vi "抓圓.vi"(0 "Image In":T2, 1 "Process":T7(ring), 2 "Optimized Mode":bool, 3 "Direction":enum16{"Inner to Outer", "Outer to Inner"}(ring), 5 "ROI":T1, 9 "Gap":i32=10 min=1 max=300, 11 "error In":errorcluster, 12 "Edge Options":T5={"Edge Polarity"=0, "Kernel Size"=3, "Width"=3, "Minimum Edge Strength"=10.0, "Interpolation Type"=enum."Bilinear Fixed", "Data Processing Method"=enum."Average"} {"Edge Polarity" items=["All Edges", "Rising Edges", "Falling Edges"]; "Minimum Edge Strength" format="%.2f"; "Width" step=2; "Kernel Size" step=2}, 13 "Point Diameter (5)":u32=5 min=3 max=1000) -> (4 "Imag e Out":T2, 6 "Line Profile":T3(graph), 10 "Gradient Information":dbl[][](graph), 14 "Ellipse":T4 {"Minor Axis"."Point 2"."Y" format="%.2f"; "Minor Axis"."Point 2"."X" format="%.2f"; "Minor Axis"."Point 1"."Y" format="%.2f"; "Minor Axis"."Point 1"."X" format="%.2f"; "Major Axis"."Point 2"."Y" format="%.2f"; "Major Axis"."Point 2"."X" format="%.2f"; "Major Axis"."Point 1"."Y" format="%.2f"; "Major Axis"."Point 1"."X" format="%.2f"; "Center"."Y" format="%.2f"; "Center"."X" format="%.2f"}, 15 "error out":errorcluster)   [LabVIEW 2015]
uses:
  <vilib>/vision/Measure.llb/Edge Options.ctl
  <vilib>/vision/Measure.llb/Edge Polarity.ctl
  <vilib>/vision/Image Controls.llb/IMAQ Image.ctl
  <vilib>/Analysis/coordinate.llb/2D Cartesian Coordinate Rotation (Scalar).vi
  <vilib>/vision/NI_Vision_Development_Module.lvlib
  <vilib>/Analysis/NI_AALPro.lvlib
panel:
  out "error out 2":errorcluster
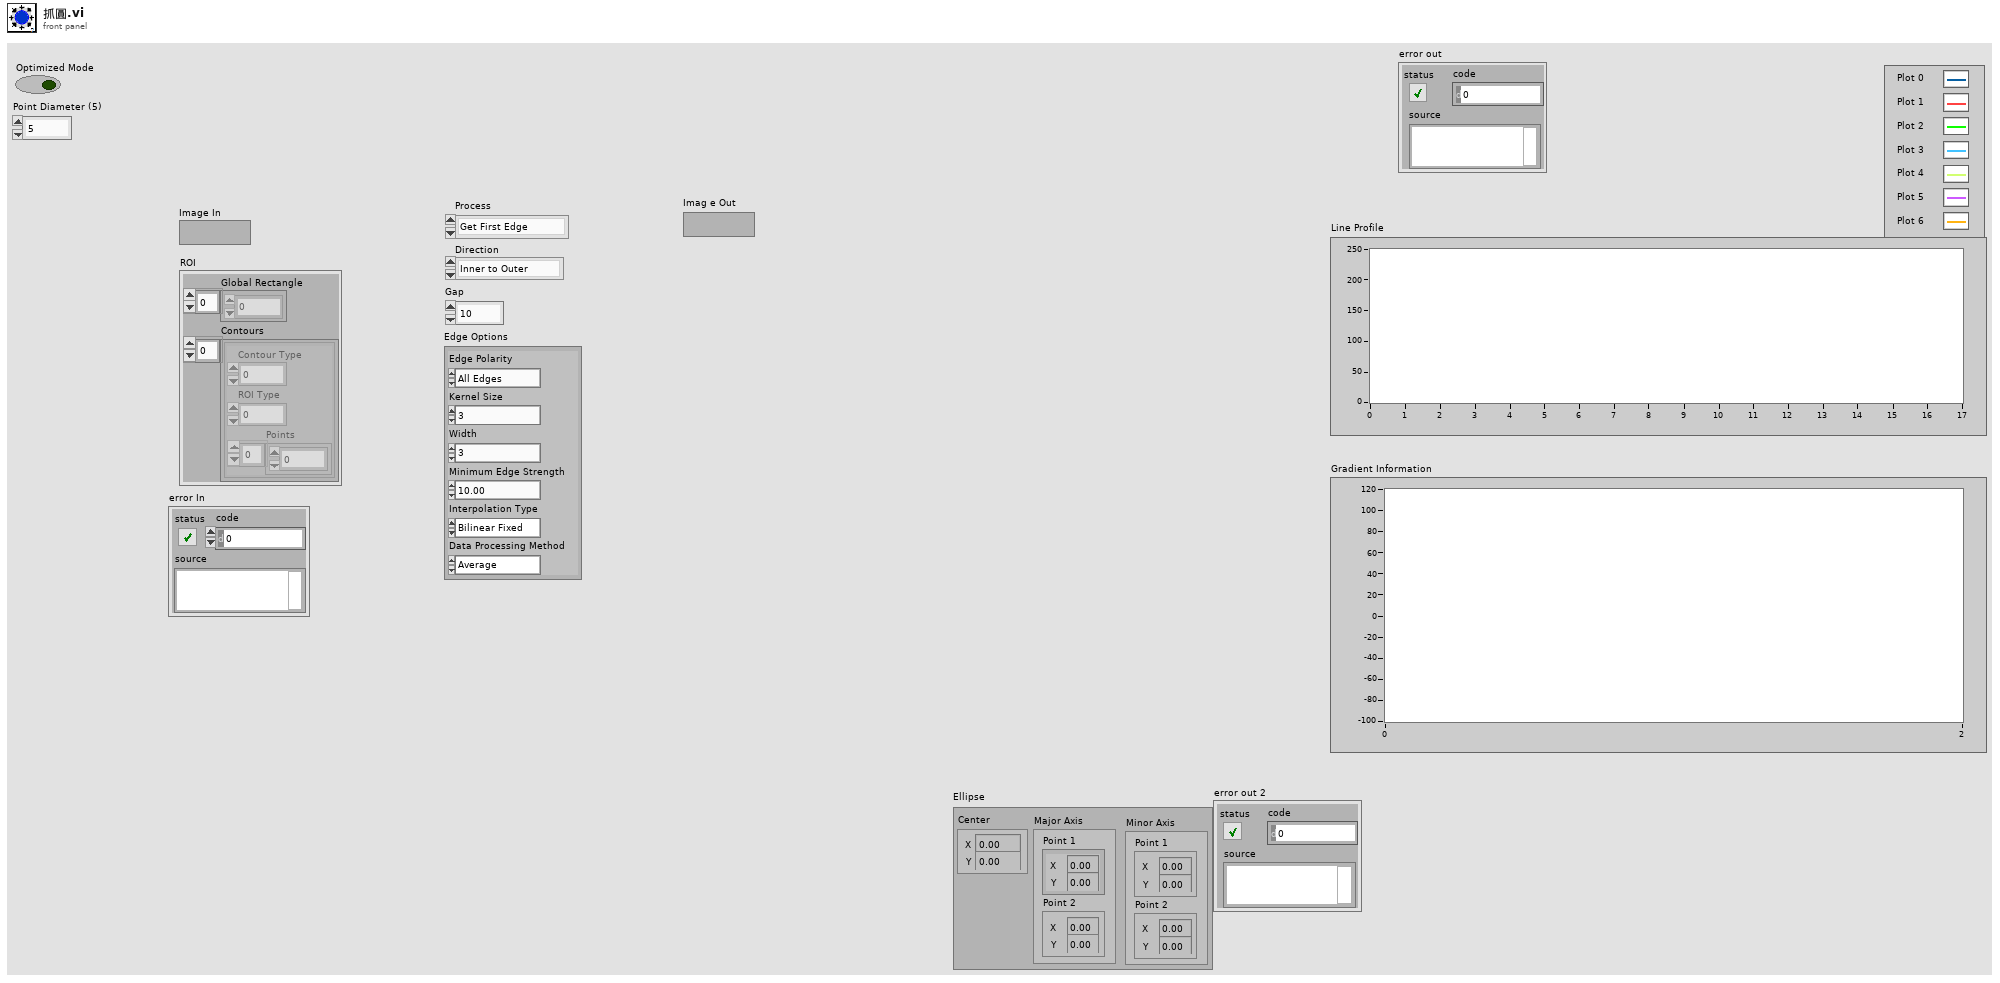
[diagram p1: front panel]
types:
  T1 = cluster{"Global Rectangle":i32[], "Contours":cluster{"Contour Type":u32, "ROI Type":u32, "Points":i32[]}[]}
  T2 = typedef "IMAQ Image.ctl" = refnum<image>
  T3 = cluster{"x0":sgl, "dx":sgl, "Pixels Line":sgl[]}[]
  T4 = cluster{"Center":cluster{"X":sgl, "Y":sgl}, "Major Axis":cluster{"Point 1":cluster{"X":sgl, "Y":sgl}, "Point 2":cluster{"X":sgl, "Y":sgl}}, "Minor Axis":cluster{"Point 1":cluster{"X":sgl, "Y":sgl}, "Point 2":cluster{"X":sgl, "Y":sgl}}}
  T5 = typedef "Edge Options.ctl" = cluster{"Edge Polarity":T6, "Kernel Size":u32, "Width":u32, "Minimum Edge Strength":sgl, "Interpolation Type":enum32{"Zero Order", "Bilinear", "Quadratic", "Cubic", "Bilinear Fixed"}, "Data Processing Method":enum32{"Average", "Median"}}
  T6 = typedef "Edge Polarity.ctl" = u32
  T7 = enum16{"Get First Edge", "Get First + Last Edge", "Get All Edges", "Get Best Edge"}
  T8 = typedef "IMAQ Point" = cluster{"X":sgl, "Y":sgl}
  T9 = typedef "IMAQ Circle" = cluster{"Center X":i32, "Center Y":i32, "Inner Radius":i32, "Outer Radius":i32, "Start Angle":dbl, "End Angle":dbl}
  T10 = cluster{"Point 1":cluster{"x":dbl, "y":dbl}, "Point 2":cluster{"x":dbl, "y":dbl}}
  T11 = typedef "IMAQ Line" = cluster{"Start X":i32, "Start Y":i32, "End X":i32, "End Y":i32}
  T12 = typedef "ROI Descriptor" = cluster{"Global Rectangle":i32[], "Contours":cluster{"ID":enum32{"External", "Internal"}, "Type":u32, "Coordinates":i32[]}[]}
  T13 = typedef "Edge New.ctl" = cluster{"Location (Pixel)":cluster{"X":sgl, "Y":sgl}, "Location (Real-World)":cluster{"X":sgl, "Y":sgl}, "Distance (Pixel)":dbl, "Distance (Real-World)":dbl, "Strength":dbl, "Noise":dbl, "Rising?":bool}
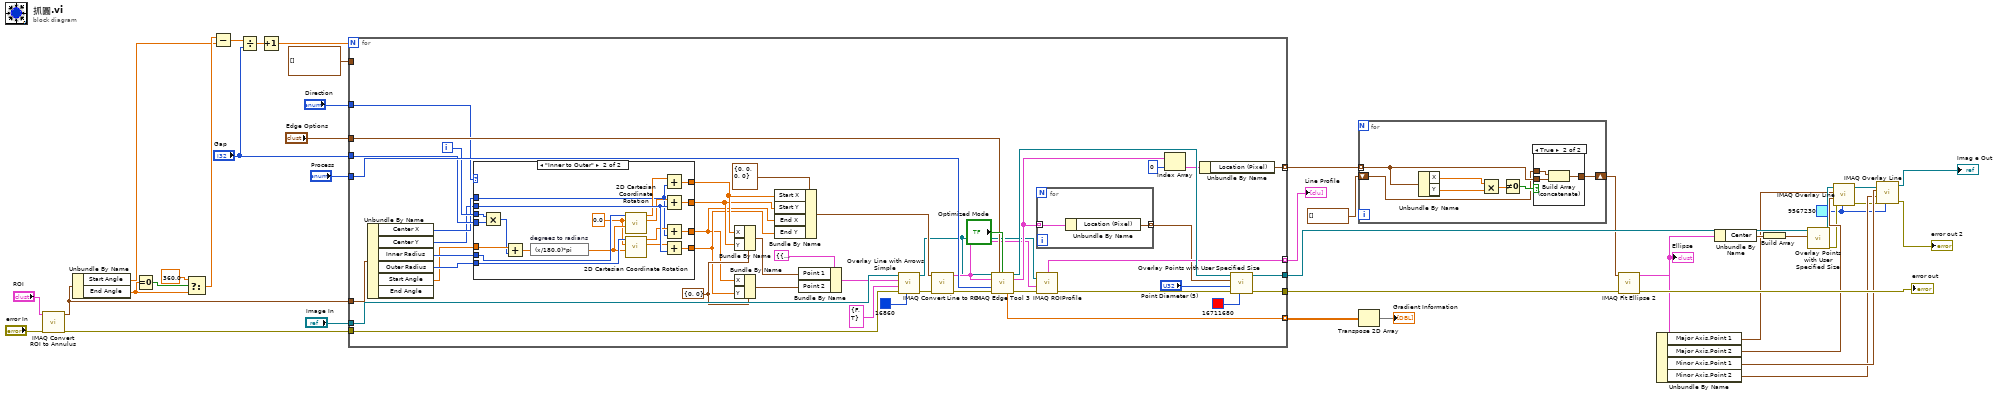
[diagram p0: block diagram]
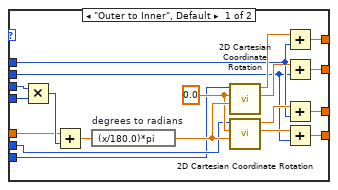
[diagram p3: hidden frame]
diagram:
  w1 = u32 9567230 ("Color")
  n1 = call "IMAQ Convert ROI to Annulus"("error in (no error)"="error In", "ROI Descriptor"="ROI") -> ("error out"=w34:errorcluster, "Annulus"=w28:T9)  [unwired: 7 in]
  n2 = Unbundle By Name(w28) -> ("Start Angle"=w18:dbl, "End Angle"=w19:dbl)
  n3 = Equal To 0?(x=w19) -> (x = 0?=w24:bool)
  n4 = Select(t=360.0, s=w24, f=w19) -> (s? t:f=w22:dbl)
  n5 = Subtract(x=w22, y=w18) -> (x-y=w21:dbl)
  n6 = Divide(x=w21, y="Gap") -> (x/y=w20:dbl)
  n7 = Increment(x=w20) -> (x+1=w35:dbl)
  n8 = for {
    N: w35 -> [_]
    tunnel: "Direction" -> [w71]
    tunnel: [w81] -> w31
    tunnel: "Image In" -> [w72]
    tunnel: w34 -> [w69]
    tunnel: [w80] -> w29
    tunnel: "Process" -> [w82]
    tunnel: "Edge Options" -> [w79]
    tunnel: [w78] -> w33 mode=indexing
    tunnel: [w77] -> w36 mode=indexing
    tunnel: [w76] -> w32 mode=indexing
    tunnel: "Gap" -> [w68]
    tunnel: w28 -> [w66]
    tunnel: T8[] [] ("Rectangle Points") -> [_]
    i -> [w67]
    w63 = cluster{"X":i32, "Y":i32} {"X"=0, "Y"=0} ("Start Point")
    n9 = Unbundle By Name(w66) -> ("Center X"=w47:i32, "Center Y"=w46:i32, "Inner Radius"=w45:i32, "Outer Radius"=w44:i32, "Start Angle"=w43:dbl)  [unwired: 1 out]
    n10 = case shown="\"Inner to Outer\"" w71 {
      tunnel: w46 -> [w89 w124]
      tunnel: w45 -> [w88 w123]
      tunnel: w44 -> [w87 w122]
      tunnel: w43 -> [w92 w121]
      tunnel: w68 -> [w90 w120]
      tunnel: w67 -> [w91 w111]
      tunnel: [w97 w106] -> w55
      tunnel: [w95 w110] -> w53
      tunnel: w47 -> [w93 w109]
      tunnel: [w94 w108] -> w52
      tunnel: [w96 w107] -> w54
      frame "Outer to Inner", Default {
        w100 = 0.0 ("y")
        n11 = Multiply(x=w91, y=w90) -> (x*y=w99:i32)
        n12 = Add(x=w92, y=w99) -> (x+y=w98:dbl)
        n13 = expression code="(x/180.0)*pi" "degrees to radians"(w98) -> (w101:dbl)
        n14 = call-poly <vilib>:"2D Cartesian Coordinate Rotation.vi"("theta"=w101, "y"=w100, "x"=w87) -> ("y out"=w104:dbl, "x out"=w105:dbl)  [unwired: 6 in, 1 out]
        n15 = call-poly <vilib>:"2D Cartesian Coordinate Rotation.vi"("theta"=w101, "y"=w100, "x"=w88) -> ("y out"=w103:dbl, "x out"=w102:dbl)  [unwired: 6 in, 1 out]
        n16 = Add(x=w105, y=w93) -> (x+y=w97:dbl)
        n17 = Add(x=w104, y=w89) -> (x+y=w96:dbl)
        n18 = Add(x=w102, y=w93) -> (x+y=w94:dbl)
        n19 = Add(x=w103, y=w89) -> (x+y=w95:dbl)
      }
      frame "Inner to Outer" {
        w114 = 0.0 ("y")
        n20 = Multiply(x=w111, y=w120) -> (x*y=w113:i32)
        n21 = Add(x=w121, y=w113) -> (x+y=w112:dbl)
        n22 = expression code="(x/180.0)*pi" "degrees to radians"(w112) -> (w115:dbl)
        n23 = call-poly <vilib>:"2D Cartesian Coordinate Rotation.vi"("theta"=w115, "y"=w114, "x"=w123) -> ("y out"=w118:dbl, "x out"=w119:dbl)  [unwired: 6 in, 1 out]
        n24 = call-poly <vilib>:"2D Cartesian Coordinate Rotation.vi"("theta"=w115, "y"=w114, "x"=w122) -> ("y out"=w117:dbl, "x out"=w116:dbl)  [unwired: 6 in, 1 out]
        n25 = Add(x=w119, y=w109) -> (x+y=w106:dbl)
        n26 = Add(x=w118, y=w124) -> (x+y=w107:dbl)
        n27 = Add(x=w116, y=w109) -> (x+y=w108:dbl)
        n28 = Add(x=w117, y=w124) -> (x+y=w110:dbl)
      }
    }
    n29 = Bundle By Name(cluster=w63, "X"=w55, "Y"=w54) -> (w61:cluster{"X":i32, "Y":i32})
    n30 = Bundle By Name(cluster=w63, "X"=w52, "Y"=w53) -> (w62:cluster{"X":i32, "Y":i32})
    n31 = Bundle By Name(cluster=T11 {"Start X"=0, "Start Y"=0, "End X"=0, "End Y"=0} ("Line"), "Start X"=w55, "Start Y"=w54, "End X"=w52, "End Y"=w53) -> (w64:T11)
    n32 = Bundle By Name(cluster=T10 {"Point 1"={"x"=50.0, "y"=50.0}, "Point 2"={"x"=70.0, "y"=70.0}} ("Line Coordinates"), "Point 1"=w61, "Point 2"=w62) -> (w58:T10)
    n33 = call "Overlay Line with Arrows Simple.vi"("Color"=u32 16860, "error in"=w69, "Arrows"=cluster{"Start point":bool, "End point":bool} {"Start point"=FALSE, "End point"=TRUE}, "Line Coordinates"=w58, "Image In"=w72) -> ("error out"=w56:errorcluster, "Image Out"=w57:T2)  [unwired: 5 in]
    n34 = call "IMAQ Convert Line to ROI"("error in (no error)"=w56, "Line"=w64) -> ("error out"=w74:errorcluster, "ROI Descriptor"=w73:T12)  [unwired: 7 in]
    n35 = call "IMAQ Edge Tool 3"("Image"=w57, "Edge Options"=w79, "Optimized Mode"="Optimized Mode", "ROI Descriptor"=w73, "Process"=w82, "error in (no error)"=w74) -> ("Image (duplicate)"=w83:T2, "Edge Information"=w86:T13[], "Gradient Values"=w77:dbl[], "error out"=w75:errorcluster)  [unwired: 5 in, 1 out]
    n36 = for {
      tunnel: w86 -> [w126] mode=indexing
      tunnel: [w125] -> w48 mode=indexing
      n37 = Unbundle By Name(w126) -> ("Location (Pixel)"=w125:cluster{"X":sgl, "Y":sgl})
    }
    n38 = call "IMAQ ROIProfile"("error in (no error)"=w75, "ROI Descriptor"=w73, "Image"=w57) -> ("error out"=w85:errorcluster, "ROI Graph"=w78:cluster{"x0":sgl, "dx":sgl, "Pixels Line":sgl[]})  [unwired: 1 in, 3 out]
    n39 = Index Array(array=w86, index=0) -> (element=w49:T13)
    n40 = Unbundle By Name(w49) -> ("Location (Pixel)"=w76:cluster{"X":sgl, "Y":sgl})
    n41 = call "Overlay Points with User Specified Size.vi"("Color"=u32 16711680, "error in"=w85, "Point Diameter (5)"="Point Diameter (5)", "Points"=w48, "Image In"=w83) -> ("error out"=w80:errorcluster, "Image Out"=w81:T2)  [unwired: 5 in]
  }
  "Line Profile" <- w33
  n42 = for {
    tunnel: w32 -> [w129] mode=indexing
    shift-right: [w128] -> w30
    shift-left: cluster{"X":sgl, "Y":sgl}[] [] -> [w127]
    n43 = Unbundle By Name(w129) -> ("X"=w133:sgl, "Y"=w132:sgl)
    n44 = Multiply(x=w133, y=w132) -> (x*y=w131:sgl)
    n45 = Not Equal To 0?(x=w131) -> (x != 0?=w130:bool)
    n46 = case shown="True" w130 {
      tunnel: w129 -> [_ w137]
      tunnel: [w134 w136] -> w128
      tunnel: w127 -> [w134 w135]
      frame False {
      }
      frame True {
        n47 = Build Array (concatenate)(w135, w137) -> (w136:cluster{"X":sgl, "Y":sgl}[])
      }
    }
  }
  n48 = Transpose 2D Array(2D array=w36) -> (transposed array=→"Gradient Information":dbl[][])
  n49 = call "IMAQ Fit Ellipse 2"("error in (no error)"=w29, "Radial Points"=w30) -> ("error out"=→"error out":errorcluster, "Ellipse"=w9:T4)  [unwired: 4 in, 4 out]
  "Ellipse" <- w9
  n50 = Unbundle By Name(w9) -> ("Major Axis.Point 1"=w8:cluster{"X":sgl, "Y":sgl}, "Major Axis.Point 2"=w7:cluster{"X":sgl, "Y":sgl}, "Minor Axis.Point 1"=w6:cluster{"X":sgl, "Y":sgl}, "Minor Axis.Point 2"=w5:cluster{"X":sgl, "Y":sgl})
  n51 = Unbundle By Name(w9) -> ("Center"=w16:cluster{"X":sgl, "Y":sgl})
  n52 = Build Array(w16) -> (w17:cluster{"X":sgl, "Y":sgl}[])
  n53 = call "Overlay Points with User Specified Size.vi"("Points"=w17, "Image In"=w31) -> ("error out"=w2:errorcluster, "Image Out"=w12:T2)  [unwired: 8 in]
  n54 = call "IMAQ Overlay Line"("Color"=w1, "error in (no error)"=w2, "End Point"=w7, "Start Point"=w8, "Image"=w12) -> ("error out"=w4:errorcluster, "Image Out"=w11:T2)  [unwired: 5 in]
  n55 = call "IMAQ Overlay Line"("Color"=w1, "error in (no error)"=w4, "End Point"=w5, "Start Point"=w6, "Image"=w11) -> ("error out"=→"error out 2":errorcluster, "Image Out"=→"Imag e Out":T2)  [unwired: 5 in]
